vi "ReadParam.vi"(8 "error in (no error)":errorcluster caption="entrée d'erreur (pas d'erreur)") -> (0 "error out":errorcluster caption="sortie d'erreur")   [LabVIEW 2020]
doc: "Lit les param et les place dans des Varglo"
uses:
  <vilib>/Utility/config.llb/Read Key (U32).vi
  ISO/Variables globales outil isospi sans MCU.vi
  <vilib>/Utility/config.llb/Read Key (Double).vi
  <vilib>/Utility/config.llb/NI_LVConfig.lvlib
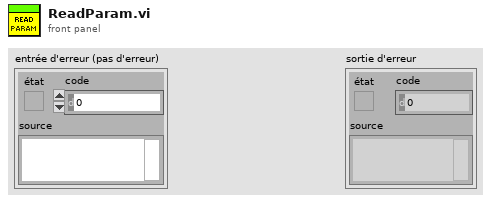
[diagram p1: front panel]
types:
  T1 = typedef "NI_LVConfig.lvlib/Config Data RefNum.ctl" = refnum<k1>
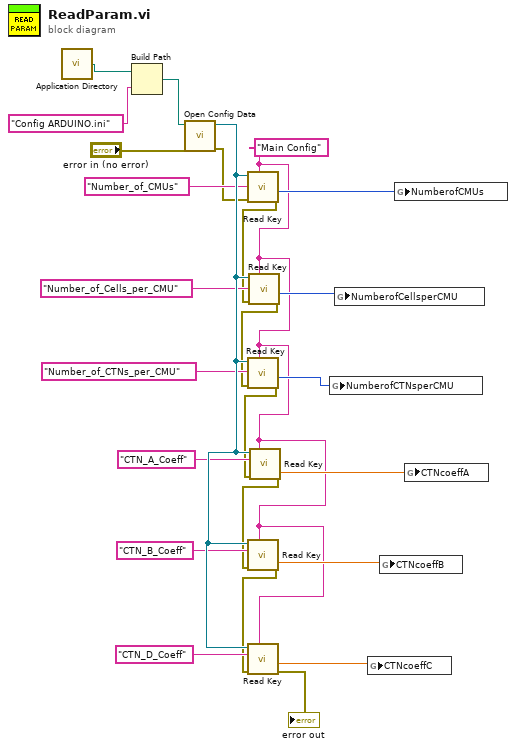
[diagram p0: block diagram]
diagram:
  w19 = "Main Config" ("section")
  n1 = call <vilib>:"Application Directory.vi"() -> ("Application Directory"=w9:path)
  n2 = Build Path(base path=w9, name or relative path="Config ARDUINO.ini") -> (appended path=w11:path)
  n3 = call <vilib>:"Open Config Data.vi"("error in (no error)"="error in (no error)", "configuration file path"=w11) -> ("error out"=w8:errorcluster, "refnum"=w18:T1)  [unwired: 7 in, 1 out]
  n4 = call-poly <vilib>:"Read Key.vi"("section"=w19, "error in (no error)"=w8, "key"="Number_of_CMUs", "refnum"=w18) -> ("error out"=w7:errorcluster, "value"=w20:u32)  [unwired: 4 in, 2 out]
  n5 = call-poly <vilib>:"Read Key.vi"("section"=w19, "error in (no error)"=w7, "key"="Number_of_Cells_per_CMU", "refnum"=w18) -> ("error out"=w6:errorcluster, "value"=w21:u32)  [unwired: 4 in, 2 out]
  n6 = call-poly <vilib>:"Read Key.vi"("section"=w19, "error in (no error)"=w6, "key"="Number_of_CTNs_per_CMU", "refnum"=w18) -> ("error out"=w5:errorcluster, "value"=w22:u32)  [unwired: 4 in, 2 out]
  n7 = call-poly <vilib>:"Read Key.vi"("section"=w19, "error in (no error)"=w5, "key"="CTN_A_Coeff", "refnum"=w18) -> ("error out"=w4:errorcluster, "value"=w23:dbl)  [unwired: 4 in, 2 out]
  n8 = call-poly <vilib>:"Read Key.vi"("section"=w19, "error in (no error)"=w4, "key"="CTN_B_Coeff", "refnum"=w18) -> ("error out"=w3:errorcluster, "value"=w24:dbl)  [unwired: 4 in, 2 out]
  n9 = call-poly <vilib>:"Read Key.vi"("section"=w19, "error in (no error)"=w3, "key"="CTN_D_Coeff", "refnum"=w18) -> ("error out"=→"error out":errorcluster, "value"=w25:dbl)  [unwired: 4 in, 2 out]
  n10 = global write "Variables globales outil isospi sans MCU.vi" "NumberofCTNsperCMU"(w22) -> ()
  n11 = global write "Variables globales outil isospi sans MCU.vi" "NumberofCellsperCMU"(w21) -> ()
  n12 = global write "Variables globales outil isospi sans MCU.vi" "CTNcoeffC"(w25) -> ()
  n13 = global write "Variables globales outil isospi sans MCU.vi" "CTNcoeffB"(w24) -> ()
  n14 = global write "Variables globales outil isospi sans MCU.vi" "NumberofCMUs"(w20) -> ()
  n15 = global write "Variables globales outil isospi sans MCU.vi" "CTNcoeffA"(w23) -> ()
